vi "dfd_2-Band Synthesis Param Validation.vi"(8 "error in (no error)":errorcluster, 9 "filter bank":T1 {"mBank_Type" items=["Uniform", "Non-Uniform"]; "mBank_Filters"."mMRate_SumWl" min=1 max=32 step=1; "mBank_Filters"."mMRate_InputIwl" min=1 max=32 step=1; "mBank_Filters"."mMRate_GainWl" min=1 max=32 step=1; "mBank_Filters"."mMRate_OutputWl" min=1 max=32 step=1; "mBank_Filters"."mMRate_InputWl" min=1 max=32 step=1; "mBank_Filters"."mMRate_CoefWl" min=1 max=32 step=1; "mBank_Filters"."mMRate_Mode" items=["Default"=-1, "No Rate Change"=0, "Interpolation"=1, "Decimation"=2, "Interpolated"=3, "Rational"=4]}, 10 "highpass channel":dbl[](array[numeric]), 11 "lowpass channel":dbl[](array[numeric])) -> (0 "error out":errorcluster, 1 "dup filter bank":T1 {"mBank_Type" items=["Uniform", "Non-Uniform"]; "mBank_Filters"."mMRate_SumWl" min=1 max=32 step=1; "mBank_Filters"."mMRate_InputIwl" min=1 max=32 step=1; "mBank_Filters"."mMRate_GainWl" min=1 max=32 step=1; "mBank_Filters"."mMRate_OutputWl" min=1 max=32 step=1; "mBank_Filters"."mMRate_InputWl" min=1 max=32 step=1; "mBank_Filters"."mMRate_CoefWl" min=1 max=32 step=1; "mBank_Filters"."mMRate_Mode" items=["Default"=-1, "No Rate Change"=0, "Interpolation"=1, "Decimation"=2, "Interpolated"=3, "Rational"=4]}, 2 "dup highpass channel":dbl[](array[numeric]), 3 "dup lowpass channel":dbl[](array[numeric]))   [LabVIEW 2017, in "NI_DigFilter_FilterBank.lvlib"]
uses:
  <vilib>/addons/Digital Filter Design/NI_DigFilter_FilterBank.lvlib
  <vilib>/addons/Digital Filter Design/FilterBank.llb/Object/DFD Bank Obj.ctl
  <vilib>/addons/Digital Filter Design/_Objects.llb/DFD Multirate Filter Obj.ctl
  <vilib>/addons/Digital Filter Design/_Objects.llb/DFD Multirate Mode.ctl
  <vilib>/addons/Digital Filter Design/_Objects.llb/DFD Coef Norm Type.ctl
  <vilib>/addons/Digital Filter Design/_Objects.llb/DFD Round-off Mode.ctl
  <vilib>/addons/Digital Filter Design/_Objects.llb/DFD FXP MRate Multiply Mode.ctl
  <vilib>/addons/Digital Filter Design/FilterBank.llb/Object/DFD Filter Bank Processing Method.ctl
  <vilib>/addons/Digital Filter Design/FilterBank.llb/Object/DFD Filter Bank Type.ctl
  <vilib>/addons/Digital Filter Design/_Misc.llb/dfd_Error Handlers (Single).vi
  <vilib>/addons/Digital Filter Design/_Misc.llb/dfd_Error Handlers (Multiple).vi
  <vilib>/addons/Digital Filter Design/NI_DigFilterLicensed.lvlib
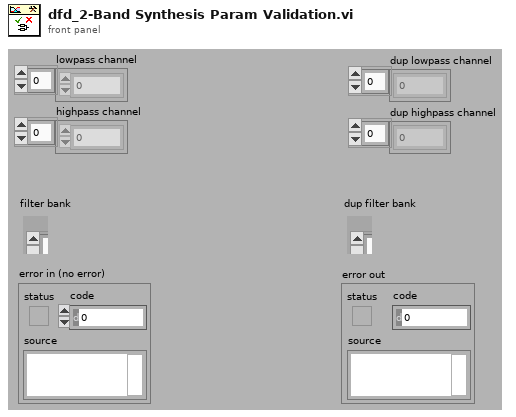
[diagram p1: front panel]
types:
  T1 = typedef "NI_DigFilter_FilterBank.lvlib/DFD Bank Obj.ctl" = cluster{"mBank_Filters":T2[], " mBank_#Bands":i32, "mBank_ProcMethod":T7, "mBank_Coeffs":dbl[], "mBank_Gain":dbl, "mBank_Type":T8}
  T2 = typedef "NI_DigFilterLicensed.lvlib/DFD Multirate Filter Obj.ctl" = cluster{"mMRate_Structure":enum16{"CIC", "FIR", "IIR", "Lattice"}, "mMRate_Mode":T3, "mMRate_Factor":i32, "mMRate_FIRParams":cluster{"mMRate_FIR_H":dbl[], "mMRate_FIR_IsNyquist?":bool, "mMRate_FIR_IsSymmetric?":bool}, "mMRate_CICParams":cluster{"mMRate_CIC_#Stage":i32, "mMRate_CIC_Lag":i32, "mMRate_CIC_Type":enum16{"Lowpass", "Highpass"}}, "mMRate_Order":i32, "mMRate_Version":string, "mMRate_Comments":string, "mMRate_RationalFactor":cluster{"mMRate_L":i32, "mMRate_M":i32}, "mMRate_Fs":dbl, "mMRate_Quantized?":bool, "mMRate_QFilterGain":dbl, "mMRate_CoefWl":i16, "mMRate_Scaling":cluster{"mMRate_ScaleByPowerOf2?":bool, "mMRate_ScaleType":T4}, "mMRate_InputWl":i16, "mMRate_OutputWl":i16, "mMRate_OutputMode":T5, "mMRate_MultMode":T6, "mMRate_BitPruning":bool, "mMRate_GainWl":i16, "mMRate_OutputFwl":i16, "mMRate_SumIwl":i16, "mMRate_InputIwl ":i16, "mMRate_SumWl":i16, "mMRate_CoefIwl":i16}
  T3 = typedef "NI_DigFilterLicensed.lvlib/DFD Multirate Mode.ctl" = i16
  T4 = typedef "NI_DigFilterLicensed.lvlib/DFD Coef Norm Type.ctl" = enum16{"No Norm", "Time Domain 1-Norm", "Time Domain 2-Norm", "Time Domain Inf-Norm"}
  T5 = typedef "NI_DigFilterLicensed.lvlib/DFD Round-off Mode.ctl" = enum16{"Nearest", "Truncation"}
  T6 = typedef "NI_DigFilterLicensed.lvlib/DFD FXP MRate Multiply Mode.ctl" = enum16{"Truncated", "Full"}
  T7 = typedef "NI_DigFilter_FilterBank.lvlib/DFD Filter Bank Processing Method.ctl" = enum16{"General", "2-Band QMF Lattice", "Cosine-Modulated"}
  T8 = typedef "NI_DigFilter_FilterBank.lvlib/DFD Filter Bank Type.ctl" = u16
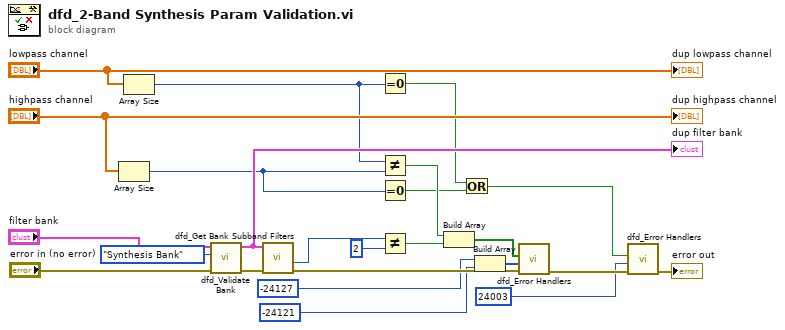
[diagram p0: block diagram]
diagram:
  n1 = Array Size(array="highpass channel") -> (size(s)=w7:i32)
  n2 = Array Size(array="lowpass channel") -> (size(s)=w8:i32)
  n3 = call <vilib>:"dfd_Validate Bank.vi"("error in (no error)"="error in (no error)", "bank type"=enum16{"Analysis Bank", "Synthesis Bank"}."Synthesis Bank", "bank in"="filter bank") -> ("error out"=w17:errorcluster, "bank out"=w18:T1)  [unwired: 6 in, 1 out]
  "dup filter bank" <- w18
  n4 = call <vilib>:"dfd_Get Bank Subband Filters.vi"("error in (no error)"=w17, "bank in"=w18) -> ("error out"=w15:errorcluster, "number of bands"=w21:i32)  [unwired: 6 in, 2 out]
  n5 = Equal To 0?(x=w8) -> (x = 0?=w5:bool)
  n6 = Not Equal?(x=w8, y=w7) -> (x != y?=w9:bool)
  n7 = Equal To 0?(x=w7) -> (x = 0?=w6:bool)
  n8 = Not Equal?(x=w21, y=2) -> (x != y?=w10:bool)
  n9 = Build Array(w9, w10) -> (w14:bool[])
  n10 = Or(x=w5, y=w6) -> (x .or. y?=w2:bool)
  n11 = Build Array(-24127 ("ERR_INVALID_SUBBAND_SIGNALS"), -24121 ("ERR_INVALID_FILTERBANK_OBJ")) -> (w11:i32[])
  n12 = call-poly <vilib>:"dfd_Error Handlers.vi"("error in (no error)"=w15, "error sources"=w11, "condition failed?"=w14) -> ("error out"=w4:errorcluster)  [unwired: 8 in]
  n13 = call-poly <vilib>:"dfd_Error Handlers.vi"("error in (no error)"=w4, "error code"=24003 ("WRN_#INPUT_ZERO"), "condition failed?"=w2) -> ("error out"=→"error out":errorcluster)  [unwired: 8 in]
  "dup lowpass channel" <- "lowpass channel"
  "dup highpass channel" <- "highpass channel"
